vi "TærningeKastBackup.vi"() -> ()   [LabVIEW 2022 SP3]
uses:
  <vilib>/numeric/Random Number (Range) U64.vi
  2e2b4b89-ef6b-4908-ba4b-1bb383d445e8.vi
  <vilib>/numeric/sub_Random U32.vi
panel:
  out "XY Graph":cluster{"Y":dbl[], "Y":dbl[]}[](graph)
  out "Sum af slag":i32
  out "sum af procent":dbl
  out "Procent array":dbl[](array[numeric])
  out "Udfalds array":i32[](array[numeric])
  in  "Andtal kast":i32
  in  "Andtal tærninger":i32
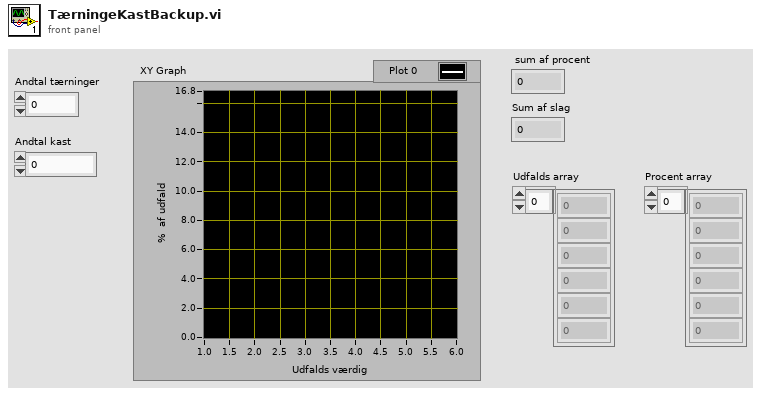
[diagram p1: front panel]
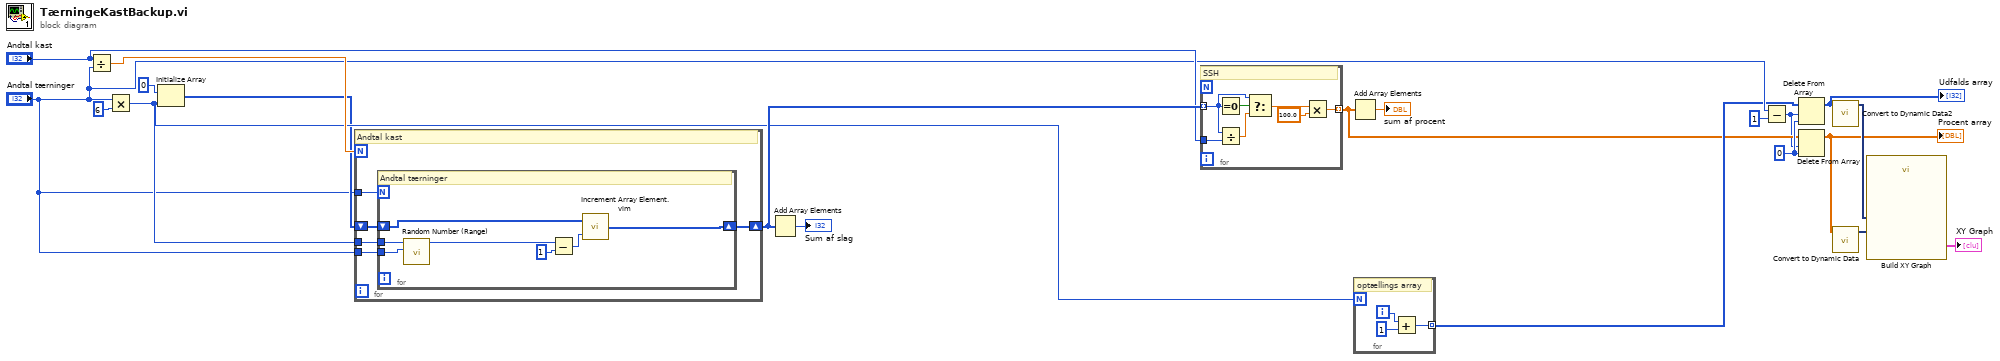
[diagram p0: block diagram]
diagram:
  w7 = 0 ("index")
  n1 = Divide(x="Andtal kast", y="Andtal tærninger") -> (x/y=w14:dbl)
  n2 = Multiply(x="Andtal tærninger", y=6) -> (x*y=w13:i32)
  n3 = Initialize Array(0 ("element"), w13) -> (w8:i32[])
  n4 = for {
    N: w14 -> [_]
    tunnel: w13 -> [w25]
    tunnel: "Andtal tærninger" -> [w24]
    tunnel: "Andtal tærninger" -> [w23]
    shift-right: [w21] -> w17
    shift-left: w8 -> [w22]
    # "Andtal kast"
    n5 = for {
      N: w23 -> [_]
      tunnel: w25 -> [w32]
      tunnel: w24 -> [w31]
      shift-right: [w26] -> w21
      shift-left: w22 -> [w28]
      # "Andtal tærninger"
      n6 = call-poly <vilib>:"Random Number (Range).vi"("lower bound (0)"=w31, "upper bound (100)"=w32) -> ("number"=w29:u64)  [unwired: 9 in]
      n7 = Subtract(x=w29, y=i64 1) -> (x-y=w27:u64)
      n8 = call "Increment Array Element.vim"("index"=w27, "array in"=w28) -> ("array out"=w26:i32[])
    }
  }
  n9 = Add Array Elements(numeric array=w17) -> (sum=→"Sum af slag":i32)
  n10 = for {
    tunnel: w17 -> [w36] mode=indexing
    tunnel: "Andtal kast" -> [w37]
    tunnel: [w33] -> w4 mode=indexing
    # "SSH"
    n11 = Equal To 0?(x=w36) -> (x = 0?=w39:bool)
    n12 = Divide(x=w36, y=w37) -> (x/y=w38:dbl)
    n13 = Select(t=w36, s=w39, f=w38) -> (s? t:f=w34:dbl)
    n14 = Multiply(x=w34, y=100.0) -> (x*y=w33:dbl)
  }
  n15 = Add Array Elements(numeric array=w4) -> (sum=→"sum af procent":dbl)
  n16 = for {
    N: w13 -> [_]
    tunnel: [w40] -> w5 mode=indexing
    i -> [w42]
    # "optællings array"
    n17 = Add(x=w42, y=1) -> (x+y=w40:i32)
  }
  n18 = Subtract(x="Andtal tærninger", y=1) -> (x-y=w3:i32)
  n19 = Delete From Array(array=w5, length=w3, index=w7) -> (array with subset deleted=w1:i32[])  [unwired: 1 out]
  "Udfalds array" <- w1
  n20 = Delete From Array(array=w4, length=w3, index=w7) -> (array with subset deleted=w2:dbl[])  [unwired: 1 out]
  "Procent array" <- w2
  n21 = call "Convert to Dynamic Data2"("Array"=w1) -> ("Dynamic Data Type"=w10:dynamicdata)  [unwired: 3 in]
  n22 = call "Convert to Dynamic Data"("Array"=w2) -> ("Dynamic Data Type"=w11:dynamicdata)  [unwired: 3 in]
  n23 = call "Build XY Graph"("Y Input"=w11, "X Input"=w10) -> ("XY Graph"=→"XY Graph":cluster{"X":dbl[], "Y":dbl[]}[])  [unwired: 8 in, 1 out]
